vi "Motor_FrictCompVol.vi"(8 "error in (no error)":errorcluster, 10 "Input Vol":dbl[](array[numeric]), 11 "Motor in":refnum<class "MotorControl.lvclass">) -> (0 "error out":errorcluster, 1 "Fric Volatage":dbl[](array[numeric]), 2 "Fric Vol + Input Vol":dbl[](array[numeric]), 3 "Motor out":refnum<class "MotorControl.lvclass">)   [LabVIEW 2015, in "MotorControl.lvclass"]
uses:
  MotorControl.lvclass
  MotorControl.lvclass/MotorControl.ctl
panel:
  in  "Enum":enum16{"Linear", "Power"}(ring)=enum."Power"
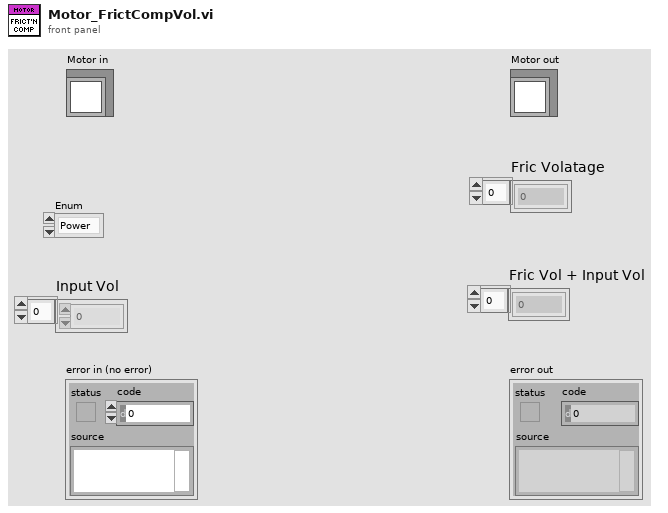
[diagram p1: front panel]
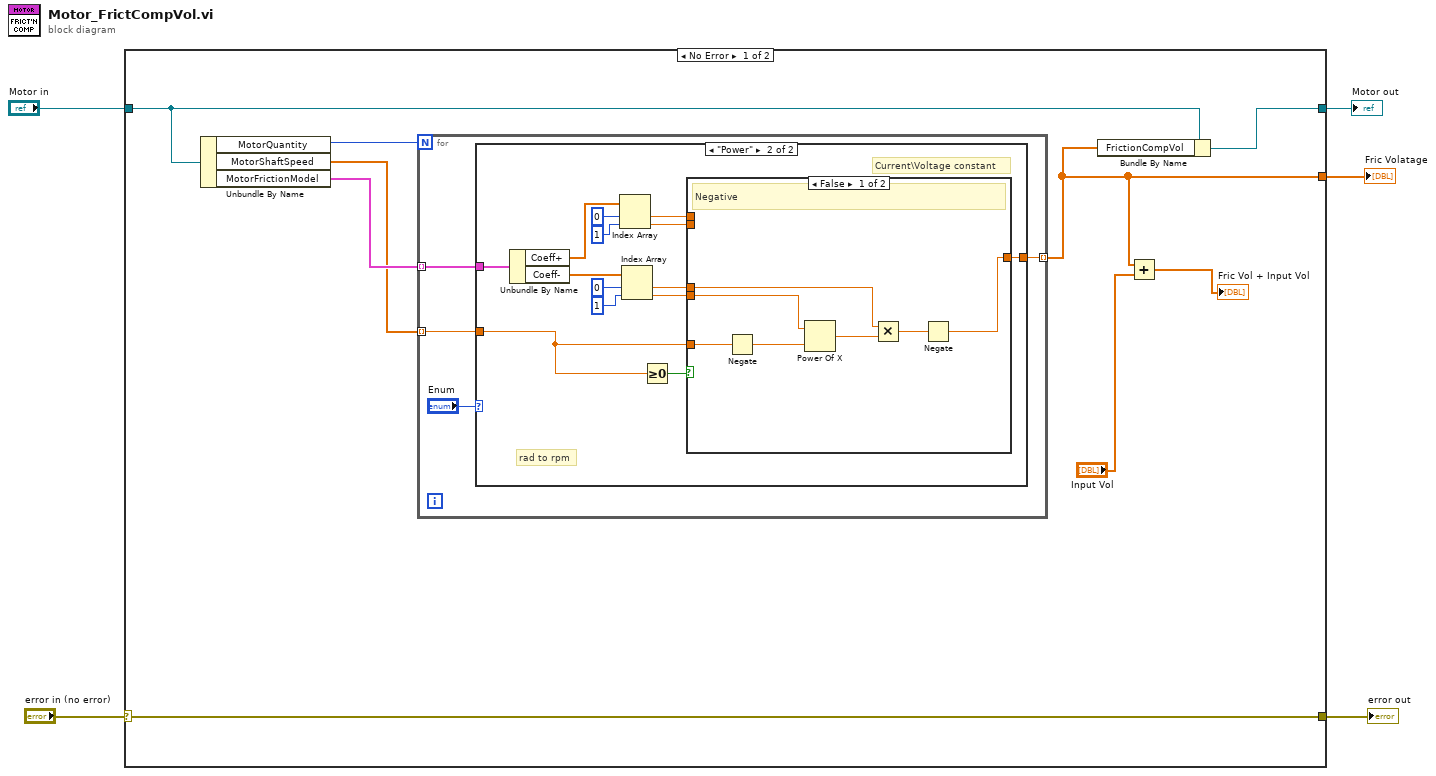
[diagram p0: block diagram]
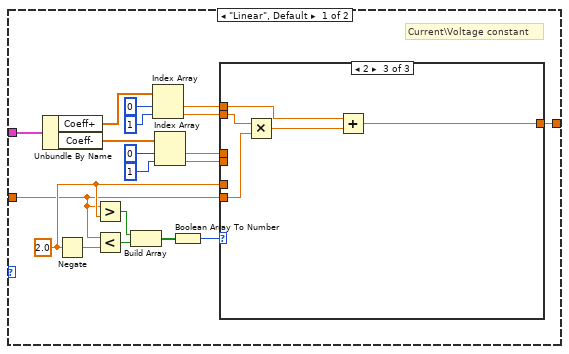
[diagram p2: hidden frame]
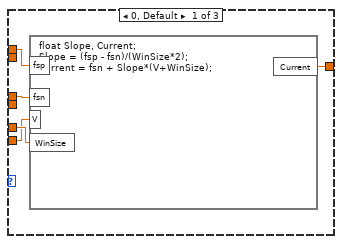
[diagram p3: hidden frame]
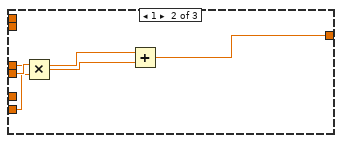
[diagram p4: hidden frame]
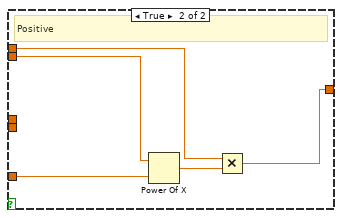
[diagram p5: hidden frame]
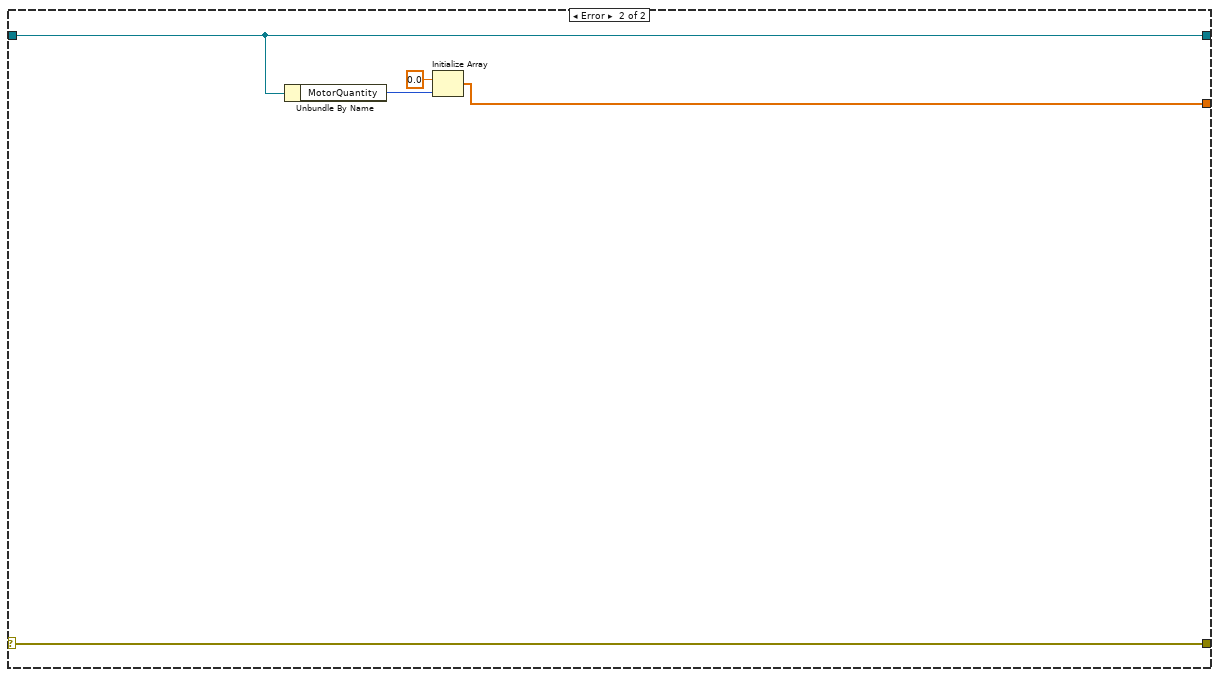
[diagram p6: hidden frame]
diagram:
  n1 = case shown="No Error" "error in (no error)" {
    selector: "error in (no error)" -> [w12 w83]
    tunnel: [w12 w83] -> w4
    tunnel: [w13 w82] -> w2
    tunnel: "Motor in" -> [w14 w82]
    tunnel: [w8 w79] -> w1
    frame No Error {
      n2 = Unbundle By Name(w14) -> ("MotorQuantity"=w11:i32, "MotorShaftSpeed"=w9:dbl[], "MotorFrictionModel"=w10:cluster{"Coeff+":dbl[], "Coeff-":dbl[]}[])
      n3 = for {
        N: w11 -> [_]
        tunnel: [w18] -> w8 mode=indexing
        tunnel: w10 -> [w17] mode=indexing
        tunnel: w9 -> [w16] mode=indexing
        n4 = case shown="\"Power\"" "Enum" {
          tunnel: [w31 w66] -> w18
          tunnel: w17 -> [w29 w65]
          tunnel: w16 -> [w30 w53]
          frame "Linear", Default {
            w37 = 2.0 ("y")
            # "Current\\Voltage constant"
            n5 = Unbundle By Name(w29) -> ("Coeff+"=w27:dbl[], "Coeff-"=w28:dbl[])
            n6 = Negate(x=w37) -> (-x=w34:dbl)
            n7 = Greater?(x=w30, y=w37) -> (0:w33:bool)
            n8 = Less?(x=w30, y=w34) -> (x < y?=w35:bool)
            n9 = Build Array(w33, w35) -> (w32:bool[])
            n10 = Index Array(array=w27, index #1=0 ("index"), index #2=1 ("index")) -> (element #1=w22:dbl, element #2=w21:dbl)
            n11 = Index Array(array=w28, index #1=0 ("index"), index #2=1 ("index")) -> (element #1=w20:dbl, element #2=w19:dbl)
            n12 = Boolean Array To Number(Boolean array=w32) -> (number=w36:u32)
            n13 = case shown="2" w36 {
              tunnel: w22 -> [w40 _ w49]
              tunnel: w20 -> [w41 w45 _]
              tunnel: w37 -> [w42 _ _]
              tunnel: w30 -> [w39 w46 w50]
              tunnel: [w38 w43 w48] -> w31
              tunnel: w19 -> [_ w47 _]
              tunnel: w21 -> [_ _ w51]
              frame 0, Default {
                n14 = formula code="float Slope, Current;\nSlope = (fsp - fsn)/(WinSize*2);\nCurrent = fsn + Slope*(V+WinSize);"("fsp"=w40, "fsn"=w41, "WinSize"=w42, "V"=w39) -> ("Current"=w38:dbl)
              }
              frame 1 {
                n15 = Multiply(x=w47, y=w46) -> (x*y=w44:dbl)
                n16 = Add(x=w45, y=w44) -> (x+y=w43:dbl)
              }
              frame 2 {
                n17 = Multiply(x=w51, y=w50) -> (x*y=w52:dbl)
                n18 = Add(x=w49, y=w52) -> (x+y=w48:dbl)
              }
            }
          }
          frame "Power" {
            # "rad to rpm"
            # "Current\\Voltage constant"
            n19 = Unbundle By Name(w65) -> ("Coeff+"=w63:dbl[], "Coeff-"=w64:dbl[])
            n20 = Index Array(array=w63, index #1=0 ("index"), index #2=1 ("index")) -> (element #1=w58:dbl, element #2=w57:dbl)
            n21 = Index Array(array=w64, index #1=0 ("index"), index #2=1 ("index")) -> (element #1=w56:dbl, element #2=w55:dbl)
            n22 = Greater Or Equal To 0?(x=w53) -> (x >= 0?=w54:bool)
            n23 = case shown="False" w54 {
              tunnel: w58 -> [_ w75]
              tunnel: w56 -> [w70 _]
              tunnel: w53 -> [w72 w78]
              tunnel: [w68 w74] -> w66
              tunnel: w55 -> [w71 _]
              tunnel: w57 -> [_ w77]
              frame False {
                # "Negative"
                n24 = Negate(x=w72) -> (-x=w67:dbl)
                n25 = Power Of X(1:w67, 2:w71) -> (0:w73:dbl)
                n26 = Multiply(x=w70, y=w73) -> (x*y=w69:dbl)
                n27 = Negate(x=w69) -> (-x=w68:dbl)
              }
              frame True {
                # "Positive"
                n28 = Power Of X(1:w78, 2:w77) -> (0:w76:dbl)
                n29 = Multiply(x=w75, y=w76) -> (x*y=w74:dbl)
              }
            }
          }
        }
      }
      n30 = Bundle By Name(cluster=w14, "FrictionCompVol"=w8) -> (w13:refnum<class "MotorControl.lvclass">)
      n31 = Add(x=w8, y="Input Vol") -> (x+y=→"Fric Vol + Input Vol":dbl[])
    }
    frame Error {
      n32 = Unbundle By Name(w82) -> ("MotorQuantity"=w81:i32)
      n33 = Initialize Array(0.0 ("element"), w81) -> (w79:dbl[])
    }
  }
  "error out" <- w4
  "Motor out" <- w2
  "Fric Volatage" <- w1
